vi "unflatten range.vi"(10 "Identifier":string, 11 "Data to Unwrap":string) -> (3 "output range":T1 {"output low" format="%.2f"; "output high" format="%.2f"})   [LabVIEW 2013, in "PID Loop.lvclass"]
uses:
  PID Loop.lvclass
  <vilib>/NI/Configuration Framework/serializable configuration/NISE_CEF_serializable configuration.lvclass
  PID Range.ctl
  String Parameters.ctl
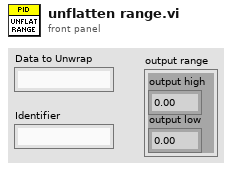
[diagram p1: front panel]
types:
  T1 = typedef "PID Loop.lvclass/PID Range.ctl" = cluster{"output high":dbl, "output low":dbl}
  T2 = typedef "PID Loop.lvclass/String Parameters.ctl" = enum16{"Setpoint", "Process Variable", "Output", "Proportional Gain", "Integral Time", "Derivative Time", "Range High", "Range Low"}
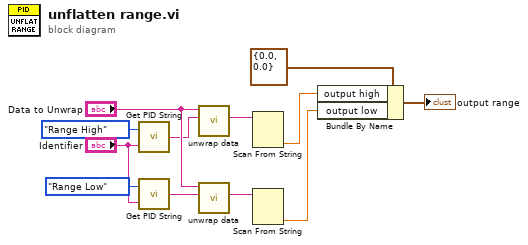
[diagram p0: block diagram]
diagram:
  n1 = call "Get PID String.vi"("PID Loop ID"="Identifier", "PID Parameter"=String_Parameters."Range High") -> ("Parameter String"=w5:string)
  n2 = call "Get PID String.vi"("PID Loop ID"="Identifier", "PID Parameter"=String_Parameters."Range Low") -> ("Parameter String"=w4:string)
  n3 = call <vilib>:"unwrap data.vi"("identifier"=w5, "data to unwrap"="Data to Unwrap") -> ("unwrapped data"=w8:string)  [unwired: 8 in, 1 out]
  n4 = call <vilib>:"unwrap data.vi"("identifier"=w4, "data to unwrap"="Data to Unwrap") -> ("unwrapped data"=w10:string)  [unwired: 8 in, 1 out]
  n5 = Scan From String(input string=w8) -> (output 1=w9:dbl)  [unwired: 4 in, 3 out]
  n6 = Scan From String(input string=w10) -> (output 1=w11:dbl)  [unwired: 4 in, 3 out]
  n7 = Bundle By Name(cluster=T1 {"output high"=0.0, "output low"=0.0} ("output range 2"), "output high"=w9, "output low"=w11) -> (→"output range":T1)
